vi "Add Default Enum.vi"(6 "Hdr Name":T1, 8 "error in (no error)":errorcluster, 9 "Enum Values":u16[](array[numeric]), 11 "Dynamic in":refnum<class "Dynamic.lvclass">) -> (0 "error out":errorcluster, 3 "Dynamic out":refnum<class "Dynamic.lvclass">)   [LabVIEW 2012, in "Measurement Channels.lvlib" / "Dynamic.lvclass"]
uses:
  Dynamic.lvclass
  Common/Controls/HeaderNames.ctl
  Class Voltage/Voltage.lvclass
  Dynamic.lvclass/Dynamic.ctl
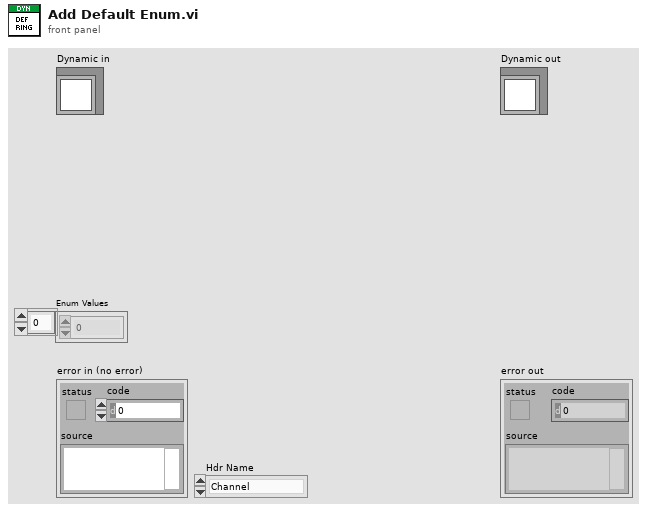
[diagram p1: front panel]
types:
  T1 = typedef "HeaderNames.ctl" = enum16{"Channel", "Device", "Spacer", "Description", "MB", "Range", "Terminal", "Coupling", "Thresh (V)", "Pulse/Rev", "Slope", "Min EU", "Min RPM", "mV/EU", "Iex", "Temp Units", "Type", "CJC Src", "CJC Val", "Ro", "Wire Cfg", "Strain Mode", "Vex", "Bridge Type", "GF", "Gauge Res", "Poisson", "Lead Res", "Init Strain", "GAF", "Scale", "Offset", "Unit (EU)", "dB?", "dB Ref", "Cal Mag", "Cal Units", "Max Temp", "Min Temp", "Max Strain", "Min Strain"}
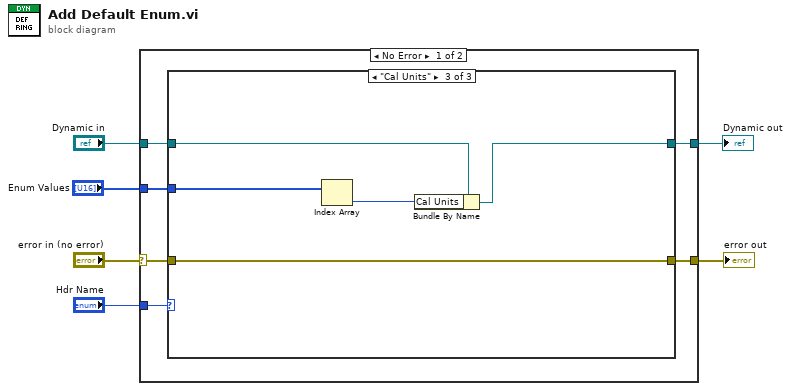
[diagram p0: block diagram]
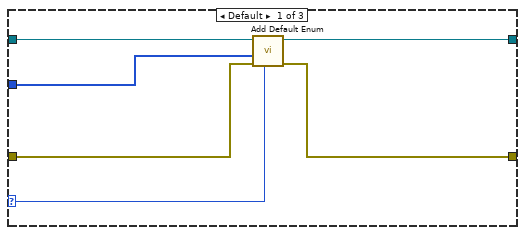
[diagram p2: hidden frame]
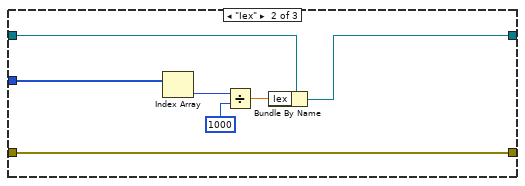
[diagram p3: hidden frame]
diagram:
  n1 = case shown="No Error" "error in (no error)" {
    selector: "error in (no error)" -> [w8 w32]
    tunnel: "Dynamic in" -> [w12 w31]
    tunnel: [w11 w31] -> w5
    tunnel: [w10 w32] -> w4
    tunnel: "Enum Values" -> [w9 _]
    tunnel: "Hdr Name" -> [w7 _]
    frame No Error {
      n2 = case shown="\"Cal Units\"" w7 {
        selector: w7 -> [w13 _ _]
        tunnel: w12 -> [w18 w22 w30]
        tunnel: [w17 w21 w29] -> w11
        tunnel: w8 -> [w16 w19 w27]
        tunnel: [w15 w19 w27] -> w10
        tunnel: w9 -> [w14 w20 w28]
        frame Default {
          n3 = call-parent "Add Default Enum.vi"("Hdr Name"=w13, "error in (no error)"=w16, "Enum Values"=w14, "Voltage in"=w18) -> ("error out"=w15:errorcluster, "Voltage out"=w17:refnum<class "Dynamic.lvclass">)  [unwired: 6 in]
        }
        frame "Iex" {
          n4 = Index Array(array=w20) -> (element=w24:u16)  [unwired: 1 in]
          n5 = Divide(x=w24, y=u16 1000) -> (x/y=w25:dbl)
          n6 = Bundle By Name(cluster=w22, "Iex"=w25) -> (w21:refnum<class "Dynamic.lvclass">)
        }
        frame "Cal Units" {
          n7 = Index Array(array=w28) -> (element=w26:u16)  [unwired: 1 in]
          n8 = Bundle By Name(cluster=w30, "Cal Units"=w26) -> (w29:refnum<class "Dynamic.lvclass">)
        }
      }
    }
    frame Error {
    }
  }
  "error out" <- w4
  "Dynamic out" <- w5
